vi "daq file read write.vi"(9 "Read(F) Write(T)":bool, 10 "Cluster":T1={"DIGITAL INPUT"={"1."="", "2."="", "3."="", "4."="", "5."="", "6."="", "7."="", "8."="", "9."="", "10."="", "11."="", "12."="", "13."="", "14."="", "15."="", "16."="", "17."="", "18."=""}, "DIGITAL OUTPUT"={"1."="", "2."="", "3."="", "4."="", "5."="", "6."="", "7."="", "8."="", "9."="", "10."="", "11."="", "12."="", "13."="", "14."=""}, "ANALOG INPUT"={"1."="", "2."="", "4"="Dev1/ai2", "3"="Dev1/ai1", "6"="Dev1/ai2", "5"="Dev1/ai1", "7"="Dev1/ai2", "8"="Dev1/ai2", "9"="Dev1/ai2", "10"="Dev1/ai2", "11"="Dev1/ai2"}, "ANALOG OUTPUT"={"1"="", "2"=""}, "Comprt"={"Leak Check Unit\nCOM Port"="", "Barcode Comport"=""}}, 11 "appended path":path) -> (0 "error out":errorcluster, 3 "Read":T1={"DIGITAL INPUT"={"1."="", "2."="", "3."="", "4."="", "5."="", "6."="", "7."="", "8."="", "9."="", "10."="", "11."="", "12."="", "13."="", "14."="", "15."="", "16."="", "17."="", "18."=""}, "DIGITAL OUTPUT"={"1."="", "2."="", "3."="", "4."="", "5."="", "6."="", "7."="", "8."="", "9."="", "10."="", "11."="", "12."="", "13."="", "14."=""}, "ANALOG INPUT"={"1."="", "2."="", "4"="Dev1/ai2", "3"="Dev1/ai1", "6"="Dev1/ai2", "5"="Dev1/ai1", "7"="Dev1/ai2", "8"="Dev1/ai2", "9"="Dev1/ai2", "10"="Dev1/ai2", "11"="Dev1/ai2"}, "ANALOG OUTPUT"={"1"="", "2"=""}, "Comprt"={"Leak Check Unit\nCOM Port"="", "Barcode Comport"=""}})   [LabVIEW 2015]
uses:
  IOs_ cluster.ctl
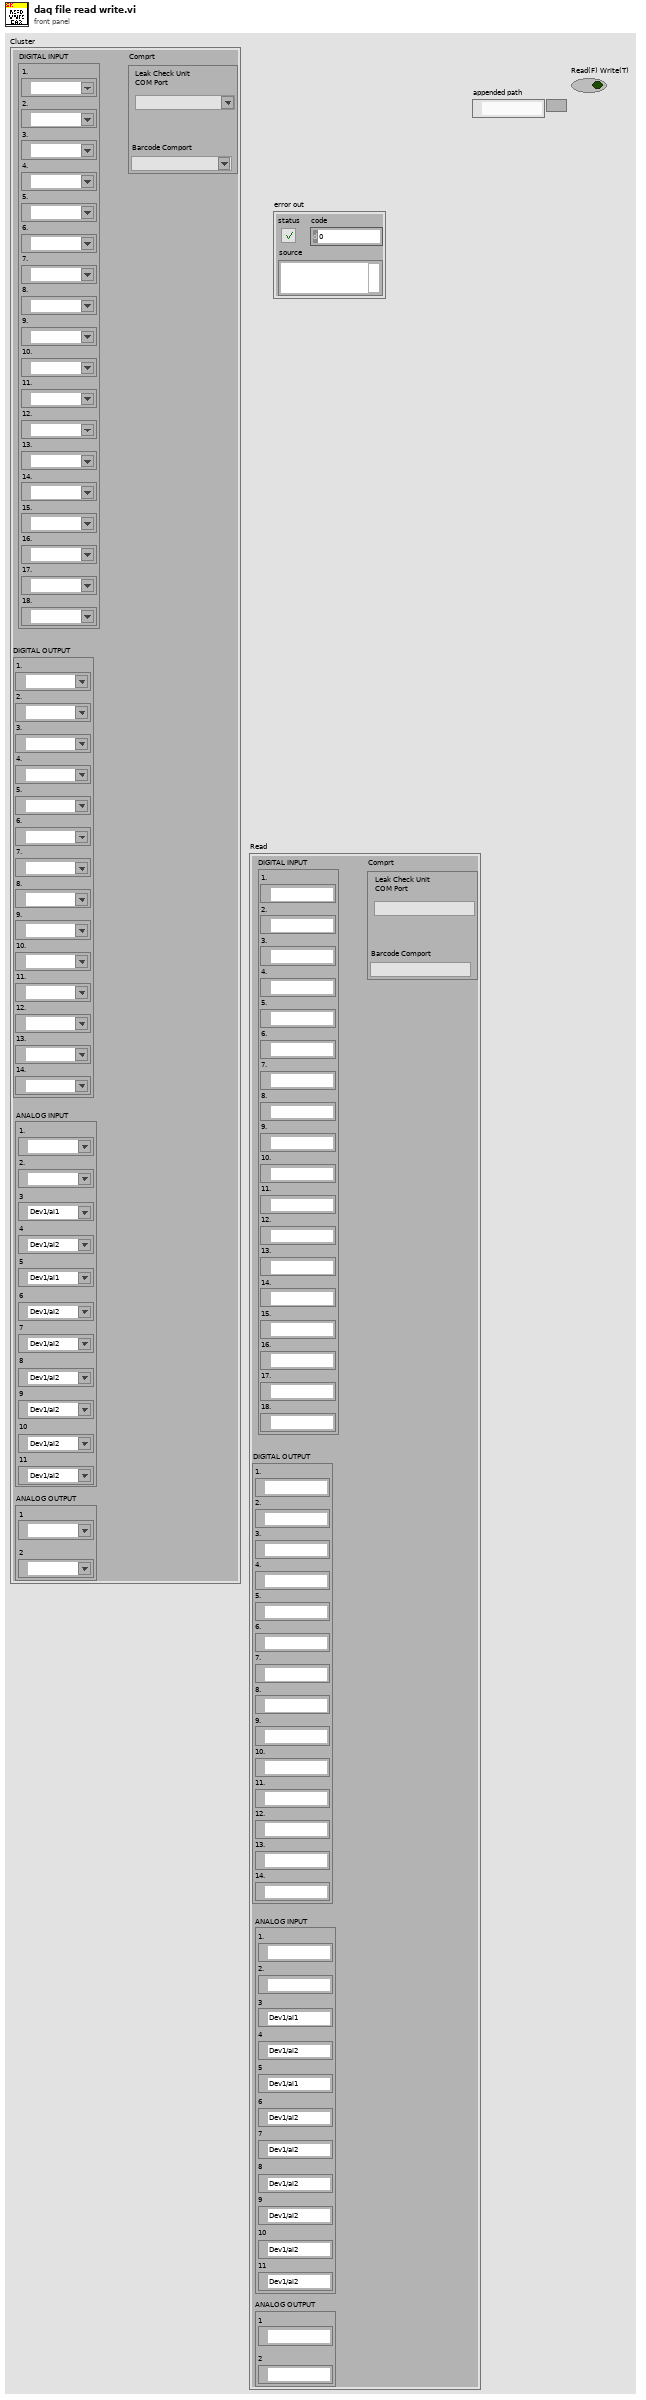
[diagram p1: front panel]
types:
  T1 = typedef "IOs_ cluster.ctl" = cluster{"DIGITAL INPUT":cluster{"1.":tag, "2.":tag, "3.":tag, "4.":tag, "5.":tag, "6.":tag, "7.":tag, "8.":tag, "9.":tag, "10.":tag, "11.":tag, "12.":tag, "13.":tag, "14.":tag, "15.":tag, "16.":tag, "17.":tag, "18.":tag}, "DIGITAL OUTPUT":cluster{"1.":tag, "2.":tag, "3.":tag, "4.":tag, "5.":tag, "6.":tag, "7.":tag, "8.":tag, "9.":tag, "10.":tag, "11.":tag, "12.":tag, "13.":tag, "14.":tag}, "ANALOG INPUT":cluster{"1.":tag, "2.":tag, "4":tag, "3":tag, "6":tag, "5":tag, "7":tag, "8":tag, "9":tag, "10":tag, "11":tag}, "ANALOG OUTPUT":cluster{"1":tag, "2":tag}, "Comprt":cluster{"Leak Check Unit\nCOM Port":refnum<visa-resource-name>, "Barcode Comport":refnum<visa-resource-name>}}
  T2 = enum16{"open", "replace", "create", "open or create", "replace or create", "replace or create with confirmation"}
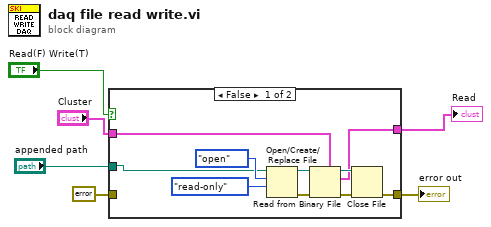
[diagram p0: block diagram]
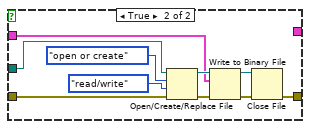
[diagram p2: hidden frame]
diagram:
  n1 = case shown="False" "Read(F) Write(T)" {
    tunnel: errorcluster {"status"=FALSE, "code"=0, "source"=""} ("error in") -> [_ w21]
    tunnel: "Cluster" -> [w12 w19]
    tunnel: [w9 w18] -> w5
    tunnel: "appended path" -> [w7 w17]
    tunnel: [w8 _] -> w1
    frame False {
      n2 = Open/Create/Replace File(file path (use dialog)=w7, operation (0:open)=T2."open", access (0:read/write)=enum16{"read/write", "read-only", "write-only"}."read-only") -> (refnum out=w13:refnum<file>, error out=w14:errorcluster)  [unwired: 3 in, 1 out]
      n3 = Read from Binary File(5:w12, 8:w14, 11:w13) -> (0:w11:errorcluster, 2:w8:T1, 3:w10:refnum<file>)  [unwired: 3 in, 1 out]
      n4 = Close File(refnum=w10, error in=w11) -> (error out=w9:errorcluster)  [unwired: 1 out]
    }
    frame True {
      n5 = Open/Create/Replace File(file path (use dialog)=w17, error in=w21, operation (0:open)=T2."open or create", access (0:read/write)=enum16{"read/write", "read-only", "write-only"}."read/write") -> (refnum out=w26:refnum<file>, error out=w25:errorcluster)  [unwired: 2 in, 1 out]
      n6 = Write to Binary File(file (use dialog)=w26, data=w19, error in=w25) -> (refnum out=w23:refnum<file>, error out=w24:errorcluster)  [unwired: 3 in, 1 out]
      n7 = Close File(refnum=w23, error in=w24) -> (error out=w18:errorcluster)  [unwired: 1 out]
    }
  }
  "error out" <- w5
  "Read" <- w1
